vi "Step Holdoff.vi"(8 "error in (no error)":errorcluster, 10 "Step up? (false)":bool, 11 "VISA resource name":refnum<visa-resource-name>) -> (0 "error out":errorcluster, 3 "VISA resource name out":refnum<visa-resource-name>, 4 "Device Errors":cluster{"code":i32, "Text":string}[](array[cluster]))   [LabVIEW 2014, in "Stanford Research DG645 - Driver.lvlib"]
doc: "Trigger Command: SPHD i\nInstrument Error Check\n\nStep trigger hold off by the current step size in the direction i. If i is true, then step up. If i is false, then step down."
uses:
  Stanford Research DG645 - Driver.lvlib
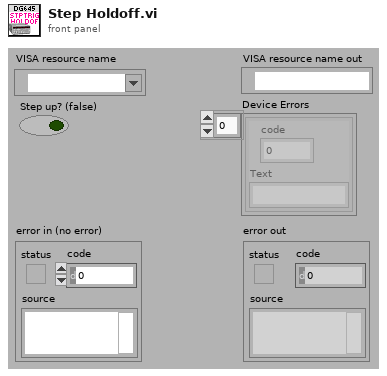
[diagram p1: front panel]
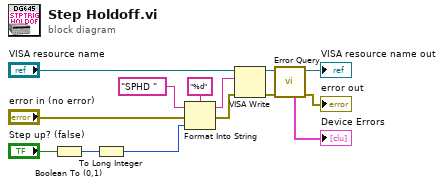
[diagram p0: block diagram]
diagram:
  n1 = Boolean To (0,1)(Boolean="Step up? (false)") -> (0, 1=w2:i16)
  n2 = To Long Integer(number=w2) -> (32bit integer=w1:i32)
  n3 = Format Into String(format string="%d", initial string="SPHD " ("command"), error in="error in (no error)", w1) -> (resulting string=w5:string, error out=w4:errorcluster)
  n4 = VISA Write(VISA resource name="VISA resource name", write buffer=w5, error in (no error)=w4) -> (VISA resource name out=w11:refnum<visa-resource-name>, error out=w8:errorcluster)  [unwired: 1 out]
  n5 = call "Error Query.vi"("error in (no error)"=w8, "VISA resource name"=w11) -> ("error out"=→"error out":errorcluster, "VISA resource name out"=→"VISA resource name out":refnum<visa-resource-name>, "Device Errors"=→"Device Errors":cluster{"code":i32, "Text":string}[])  [unwired: 7 in]
